vi "main(backup180705).vi"() -> ()   [LabVIEW 2018]
panel:
  in  "Controls Tabs":enum32{"Fire Operations", "Manual Operations"}(tab)
  in  "Fire Button":bool
  in  "Abort Button":bool
  in  "Fire Checklist":bool[](array[boolean])
  in  "ARM":bool
  out "ARM Indicator":bool
  in  "Pressurize":bool
  out "ARM Indicator 2":bool
  out "Countdown":dbl
  in  "NC-P":bool
  out "NC-P Status":bool
  in  "Actuate":bool
  in  "NO-P":bool
  out "NO-P Status":bool
  in  "NC-F":bool
  out "NC-F Status":bool
  in  "NC-FI":bool
  out "NC-FI Status":bool
  in  "NC-FP":bool
  out "NC-FP Status":bool
  in  "NC-O":bool
  out "NC-O Status":bool
  in  "NC-OI":bool
  out "NC-OI Status":bool
  in  "NC-OP":bool
  out "NC-OP Status":bool
  in  "Safety":bool
  in  "Ignition\nTest":bool
  in  "Pump":bool
  out "Fill Timer":dbl
  in  "Reset Timer":bool
  in  "Fill Progress":dbl(slide) scale=0.0..10.0
  in  "Time Target":dbl
  in  "Ignition Type (Testing)":u16(ring)
  in  "Fire Sequence Tabs":T1(tab)
  in  "NC-F\nTiming":cluster{dbl, dbl, dbl, dbl, dbl, dbl}(slide) scale=0.0..10.0
  in  "NC-O\nTiming":cluster{dbl, dbl, dbl, dbl, dbl, dbl}(slide) scale=0.0..10.0
  in  "Ignitor\nTiming":cluster{dbl, dbl, dbl, dbl, dbl, dbl}(slide) scale=0.0..10.0
  in  "NC-FI\nTiming":cluster{dbl, dbl, dbl, dbl, dbl, dbl}(slide) scale=0.0..10.0
  in  "NC-OI\nTiming":cluster{dbl, dbl, dbl, dbl, dbl, dbl}(slide) scale=0.0..10.0
  in  "Fire\nTiming":cluster{dbl, dbl, dbl}(slide) scale=0.0..10.0
  in  "NC-F Invert":bool
  in  "NC-O Invert":bool
  in  "Ignitor Invert":bool
  in  "NC-FI Invert":bool
  in  "NC-OI Invert":bool
  in  "Ignition Type":u16(ring)
  in  "Countdown + Fring\nLength":dbl
  in  "NC-F Open Delay":dbl
  in  "NC-O Open Delay":dbl
  in  "NC-FI Open Delay":dbl
  in  "Igniter Active Delay":dbl
  in  "NC-OI Open Delay":dbl
  in  "NC-F Close Delay":dbl
  in  "NC-O Close Delay":dbl
  in  "NC-FI Close Delay":dbl
  in  "Igniter Inactive Delay":dbl
  in  "NC-OI Close Delay":dbl
  in  "Edit Fire \nSequence":bool
  in  "SAFE State":bool[](array[boolean])
  in  "ARMED State":bool[](array[boolean])
  in  "Pressurized\nState":bool[](array[boolean])
  in  "Post-Fire\nState":bool[](array[boolean])
  out "Post-Fire\nIndicator":bool
  out "Pressurized Indicator":bool
  out "Pressurized Indicator 2":bool
  out "Pressurized Indicator 3":bool
  # "Verify BOTH PANELS\nof the firing sequence\nare correctly configured"
  # "Verify all sensors readings\nare within acceptable\noperating conditions"
  # "Verify PA system is\noperational and range\nadmin is notified"
  # "Verify range is clear"
  # "Go/No go"
  # "Invert"
  # "Start"
  # "End"
  # "Countdown\nLength"
  # "Fire State"
  # "NC-P"
  # "Hardware Delays"
  # "Opening"
  # "Closing"
  # "NO-P"
  # "NC-F"
  # "NC-O"
  # "NC-F"
  # "Igniter"
  # "NC-FI"
  # "NC-FI"
  # "NC-OI"
  # "NC-O"
  # "NC-OI"
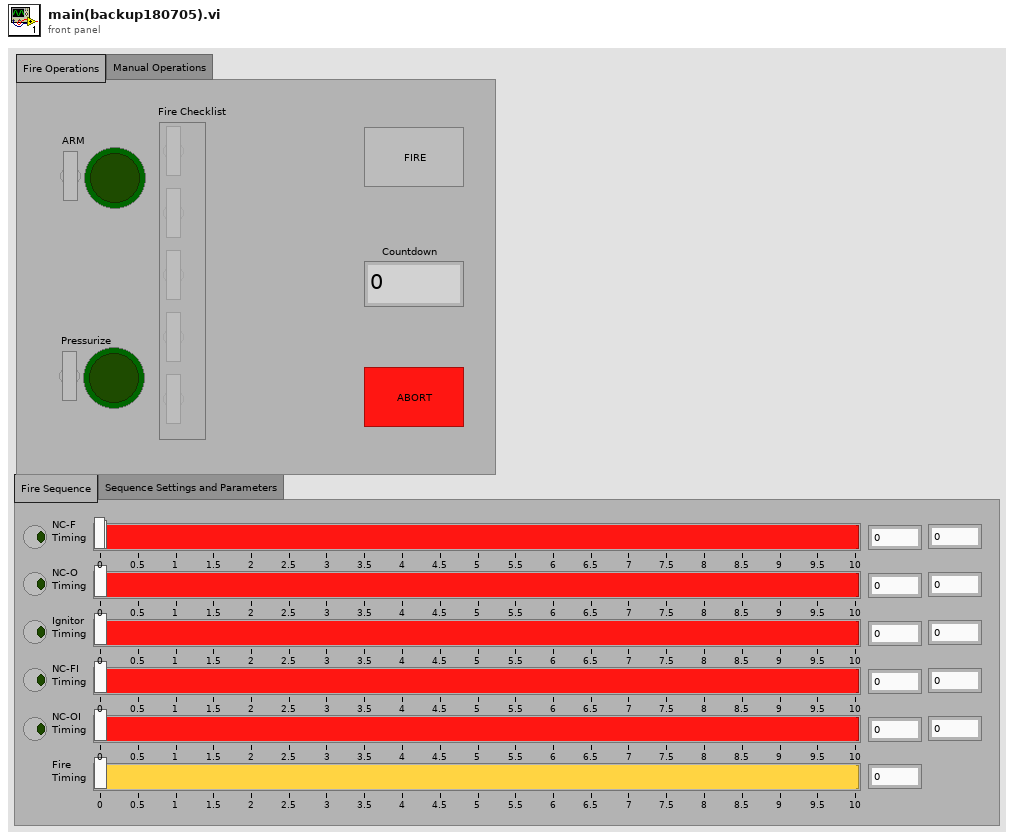
[diagram p1: front panel]
types:
  T1 = enum32{"Fire Sequence", "Sequence Settings and Parameters"}
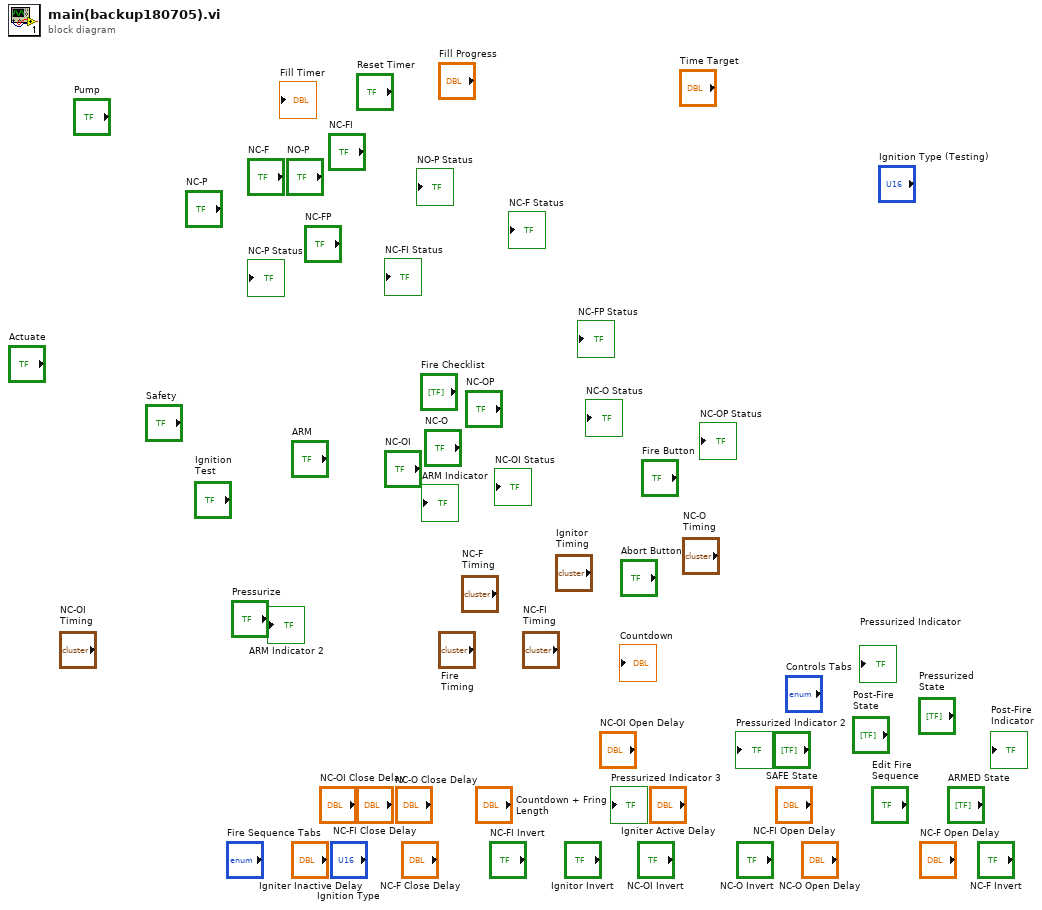
[diagram p0: block diagram]
diagram:
